vi "Clean_up_SW_Tree.vi"() -> ()   [LabVIEW 2010]
panel:
  out "Files Removed to:":path
  out "No of Removed files":i32
  out "Removed filename":string
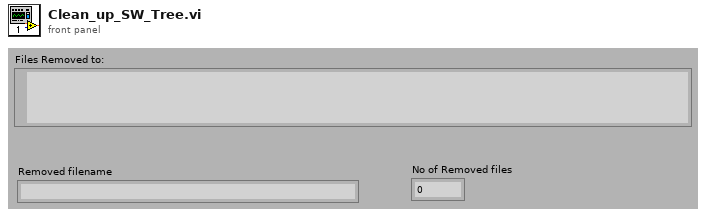
[diagram p1: front panel]
types:
  T1 = cluster{"second":i32, "minute":i32, "hour":i32, "day of month":i32, "month":i32, "year":i32, "day of week":i32, "day of year":i32, "is DST":i32}
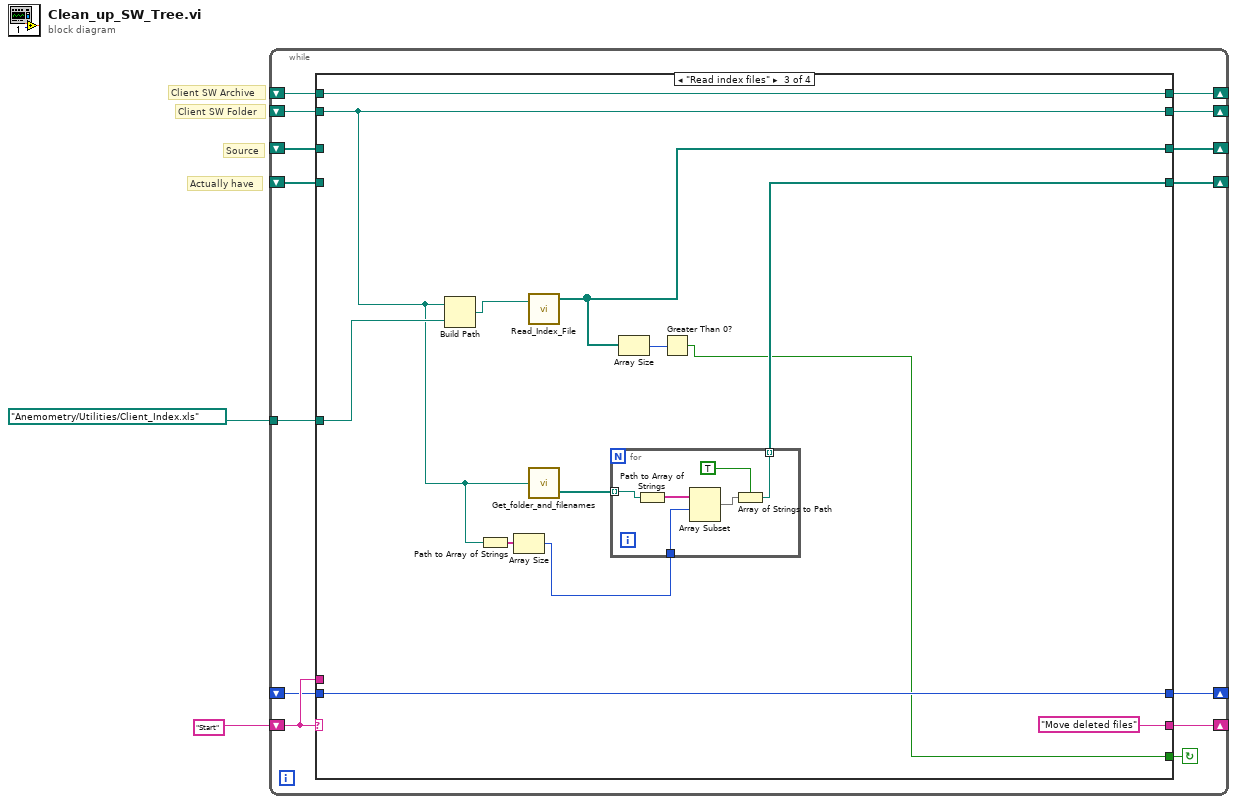
[diagram p0: block diagram]
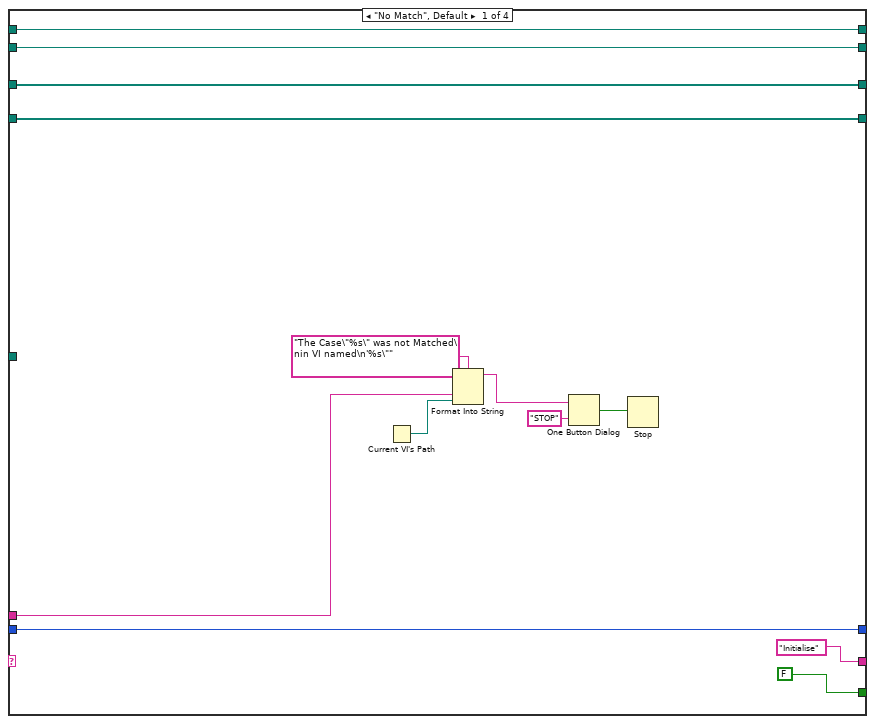
[diagram p2: hidden frame]
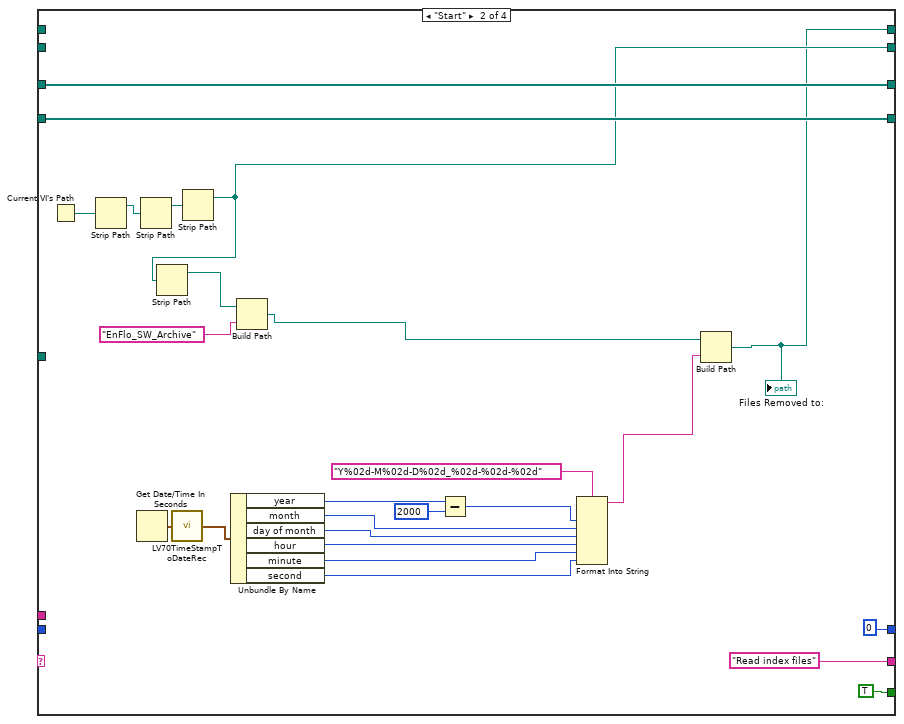
[diagram p3: hidden frame]
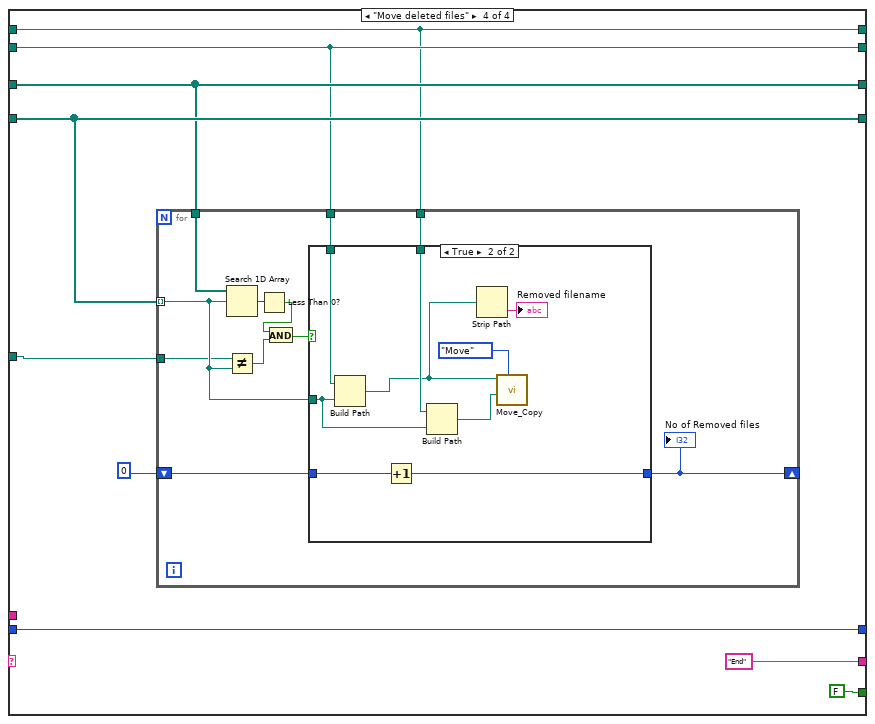
[diagram p4: hidden frame]
diagram:
  # "Actually have"
  # "Source"
  # "Client SW Archive"
  # "Client SW Folder"
  n1 = while {
    shift-left: "Start" -> [w14]
    shift-right: [w15] -> _
    shift-right: [w11] -> _
    shift-left: _ -> [w12]
    shift-right: [w9] -> _
    shift-left: _ -> [w10]
    shift-right: [w6] -> _
    shift-left: _ -> [w4]
    shift-right: [w13] -> _
    shift-left: _ -> [w8]
    shift-right: [w7] -> _
    shift-left: _ -> [w5]
    tunnel: path "Anemometry/Utilities/Client_Index.xls" -> [w3]
    stop <- w16 continue-if-true
    n2 = case shown="\"Read index files\"" w14 {
      tunnel: [FALSE TRUE w55 FALSE] -> w16
      tunnel: ["Initialise" "Read index files" "Move deleted files" "End"] -> w15
      tunnel: w14 -> [w24 _ _ _]
      tunnel: [w21 w49 w60 w77] -> w13
      tunnel: w12 -> [w20 w51 _ w78]
      tunnel: [w20 w51 w62 w78] -> w11
      tunnel: w10 -> [w19 w50 _ w79]
      tunnel: [w19 w50 w56 w79] -> w9
      tunnel: w8 -> [w21 _ w60 w77]
      tunnel: [w18 w45 w63 w76] -> w7
      tunnel: [w17 0 w66 w80] -> w6
      tunnel: w5 -> [w18 _ w63 w76]
      tunnel: w4 -> [w17 _ w66 w80]
      tunnel: w3 -> [_ _ w65 w74]
      frame "No Match", Default {
        n3 = Current VI's Path() -> (path=w23:path)
        n4 = Format Into String(format string="The Case\"%s\" was not Matched\nin VI named\n'%s\"" ("Format String"), w24, w23) -> (resulting string=w27:string)  [unwired: 2 in, 1 out]
        n5 = One Button Dialog(message=w27, button name ("OK")="STOP") -> (true=w25:bool)
        n6 = Stop(stop? (T)=w25) -> ()
      }
      frame "Start" {
        n7 = Current VI's Path() -> (path=w52:path)
        n8 = Strip Path(path=w52) -> (stripped path=w43:path)  [unwired: 1 out]
        n9 = Get Date/Time In Seconds() -> (seconds since 1Jan1904=w30:timestamp)
        n10 = Strip Path(path=w43) -> (stripped path=w42:path)  [unwired: 1 out]
        n11 = call <vilib>:"LV70TimeStampToDateRec.vi"("time stamp"=w30) -> ("date time rec"=w32:T1)
        n12 = Strip Path(path=w42) -> (stripped path=w49:path)  [unwired: 1 out]
        n13 = Strip Path(path=w49) -> (stripped path=w48:path)  [unwired: 1 out]
        n14 = Unbundle By Name(w32) -> ("year"=w40:i32, "month"=w36:i32, "day of month"=w35:i32, "hour"=w34:i32, "minute"=w33:i32, "second"=w41:i32)
        n15 = Build Path(base path=w48, name or relative path="EnFlo_SW_Archive") -> (appended path=w46:path)
        n16 = Subtract(x=w40, y=2000) -> (x-y=w38:i32)
        n17 = Format Into String(format string="Y%02d-M%02d-D%02d_%02d-%02d-%02d", w38, w36, w35, w34, w33, w41) -> (resulting string=w31:string)  [unwired: 2 in, 1 out]
        n18 = Build Path(base path=w46, name or relative path=w31) -> (appended path=w45:path)
        "Files Removed to:" <- w45
      }
      frame "Read index files" {
        n19 = Build Path(base path=w60, name or relative path=w65) -> (appended path=w64:path)
        n20 = Path to Array of Strings(0:w60) -> (2:w58:string[])  [unwired: 1 out]
        n21 = Array Size(array=w58) -> (size(s)=w57:i32)
        n22 = call "Read_Index_File.vi"("Index Filename"=w64) -> ("Filenames"=w62:path[])  [unwired: 1 in, 2 out]
        n23 = call "Get_folder_and_filenames.vi"("file path (dialog if empty)"=w60) -> ("Files"=w59:path[])  [unwired: 1 out]
        n24 = for {
          tunnel: w59 -> [w73] mode=indexing
          tunnel: w57 -> [w71]
          tunnel: [w69] -> w56 mode=indexing
          n25 = Path to Array of Strings(0:w73) -> (2:w72:string[])  [unwired: 1 out]
          n26 = Array Subset(array=w72, index=w71) -> (w70:string[])  [unwired: 1 in]
          n27 = Array of Strings to Path(0:w70, 1:TRUE ("relative")) -> (2:w69:path)
        }
        n28 = Array Size(array=w62) -> (size(s)=w61:i32)
        n29 = Greater Than 0?(x=w61) -> (x > 0?=w55:bool)
      }
      frame "Move deleted files" {
        n30 = for {
          tunnel: w79 -> [w88] mode=indexing
          tunnel: w78 -> [w93]
          tunnel: w77 -> [w92]
          tunnel: w76 -> [w91]
          shift-right: [w89] -> _
          shift-left: 0 -> [w90]
          tunnel: w74 -> [w87]
          n31 = Search 1D Array(1D array=w93, element=w88) -> (index of element=w86:i32)  [unwired: 1 in]
          n32 = Not Equal?(x=w87, y=w88) -> (x != y?=w85:bool)
          n33 = Less Than 0?(x=w86) -> (x < 0?=w84:bool)
          n34 = And(x=w84, y=w85) -> (x .and. y?=w83:bool)
          n35 = case shown="True" w83 {
            tunnel: w92 -> [_ w101]
            tunnel: w91 -> [_ w100]
            tunnel: w88 -> [_ w99]
            tunnel: w90 -> [w94 w96]
            tunnel: [w94 w95] -> w89
            frame False {
            }
            frame True {
              n36 = Build Path(base path=w101, name or relative path=w99) -> (appended path=w98:path)
              n37 = Increment(x=w96) -> (x+1=w95:i32)
              n38 = Build Path(base path=w100, name or relative path=w99) -> (appended path=w102:path)
              n39 = Strip Path(path=w98) -> (name=→"Removed filename":string)  [unwired: 1 out]
              n40 = call "Move_Copy.vi"("Mode"=enum16{"Move", "Copy"}."Move", "target path"=w102, "source path"=w98) -> ()  [unwired: 4 in]
            }
          }
          "No of Removed files" <- w89
        }
      }
    }
  }
